vi "CreatMessageEvent.vi"(0 "object in":refnum<class "Application.lvclass">, 5 "error in (no error)":errorcluster) -> (14 "object out":refnum<class "Application.lvclass">, 19 "error out":errorcluster)   [LabVIEW 2019, in "Application.lvclass"]
uses:
  Application.lvclass
  Application.lvclass/Application.ctl
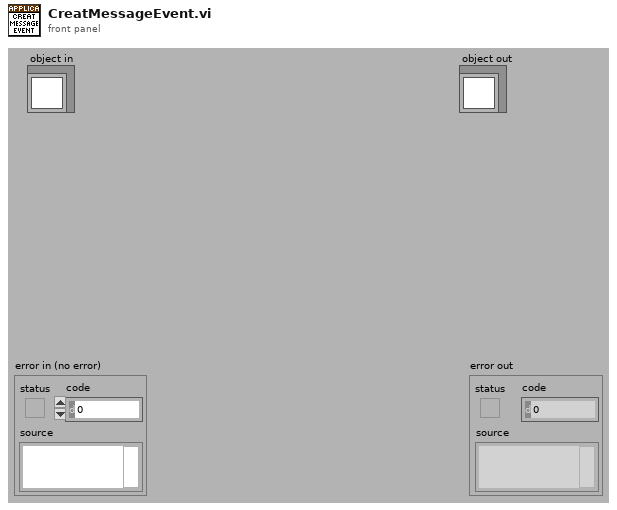
[diagram p1: front panel]
types:
  T1 = cluster{"Message":string, "Message Data":variant}
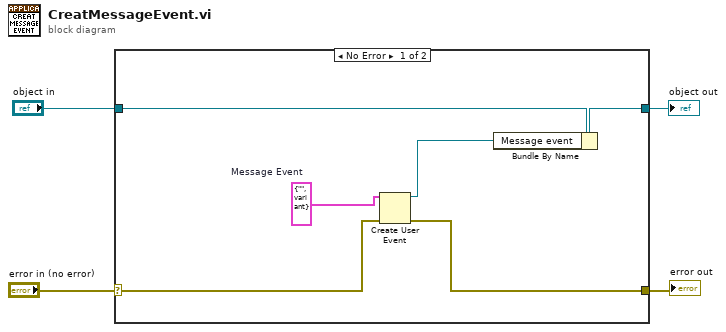
[diagram p0: block diagram]
diagram:
  n1 = case shown="No Error" "error in (no error)" {
    selector: "error in (no error)" -> [w10 w12]
    tunnel: [w9 w12] -> w3
    tunnel: [w6 w11] -> w1
    tunnel: "object in" -> [w7 w11]
    frame No Error {
      w8 = T1 {"Message"="", "Message Data"=variant}  # Message Event
      n2 = Create User Event(user event datatype=w8, error in=w10) -> (user event=w5:refnum<user-event>, error out=w9:errorcluster)
      n3 = Bundle By Name(cluster=w7, "Message event"=w5) -> (w6:refnum<class "Application.lvclass">)
    }
    frame Error {
    }
  }
  "error out" <- w3
  "object out" <- w1
